vi "ArrDevMeasAction.vi"(6 "Scan":bool, 7 "DevId":i32, 8 "error in (no error)":errorcluster caption="entrée d'erreur (pas d'erreur)", 9 "CurvePointIndex":i32, 10 "AllPointIndex":i32, 11 "Device In":refnum<class "AndorSpectro.lvclass"> caption="DNL_LabVIEW Object in") -> (0 "error out":errorcluster caption="sortie d'erreur", 1 "ArrDevDat":T1[](array[typedef]), 2 "ArrDevDatOut":dbl[][](array[numeric]), 3 "Device Out":refnum<class "AndorSpectro.lvclass"> caption="DNL_LabVIEW Object out", 5 "MeasOut":dbl[](array[numeric]))   [LabVIEW 2019, in "AndorSpectro.lvclass"]
uses:
  AndorSpectro.lvclass
  C:/Programmes Labview/LabscanV1A/DevicesClass/BaseDevice/BaseDevice.lvclass
  Experiment Class/ArrDevData.ctl
  AndorSpectro.lvclass/AndorSpectro.ctl
  BaseDevice/BaseDevice.lvclass/BaseDevice.ctl
  <userlib>/ATSpectrograph/GUI/AndorNoiseCorr.ctl
  BaseDevice/Accessor/GetBaseDataPath.vi
  <userlib>/GenProg/ReadValByRefVariant.vi
  <userlib>/GenProg/ReadbyWeakRefBool.vi
  <userlib>/GenProg/ReadValByRefBool.vi
  <userlib>/GenProg/ReadValByRefDblArr.vi
  <userlib>/GenProg/ReadValByRefI32Arr2D.vi
panel:
  out "ControlsNames":string[](array[string])
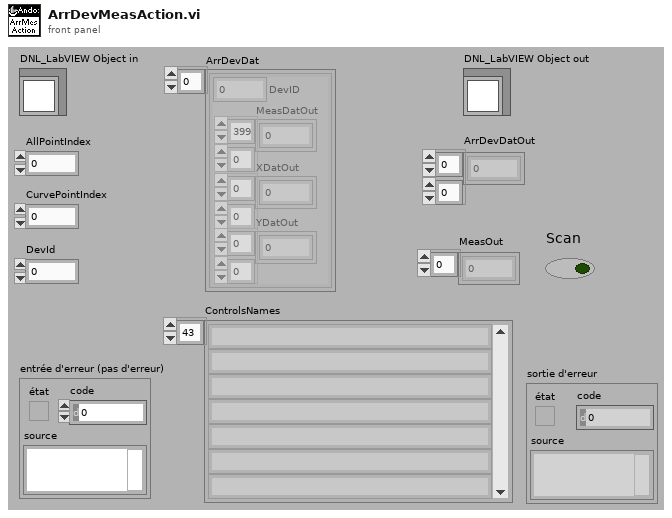
[diagram p1: front panel]
types:
  T1 = typedef "ArrDevData.ctl" = cluster{"MeasDatOut":dbl[][], "XDatOut":dbl[][], "YDatOut":dbl[][], "DevID":i32}
  T2 = typedef "AndorNoiseCorr.ctl" = enum16{"Off", "Selected Curve", "One For Every Acq"}
  T3 = cluster{"WB Start":i32, "WB End":i32, "Active":bool}[]
  T4 = cluster{"Message":string, "Data":variant, "Code":i32}
  T5 = typedef "AndorSpectro.lvclass/AndorSpectro_Func.ctl" = enum16{"ReadSpectrum (cnt)", "SetWavelenght (nm)"}
  T6 = cluster{"Scan":bool, "CurvePointIndex":i32, bool}
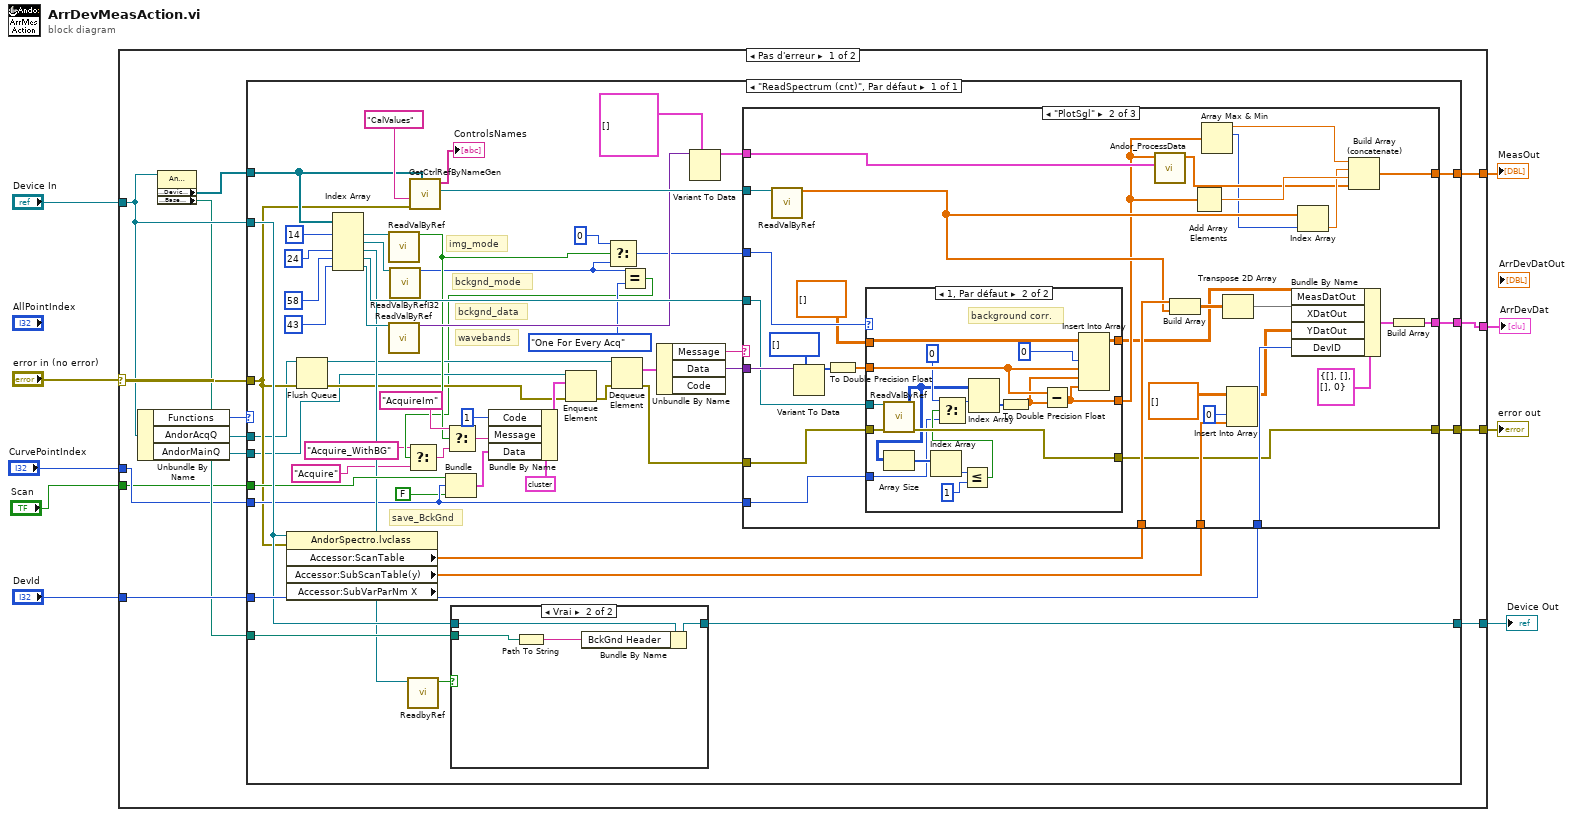
[diagram p0: block diagram]
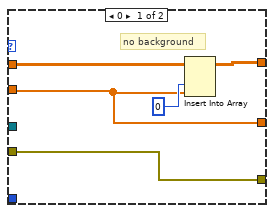
[diagram p4: hidden frame]
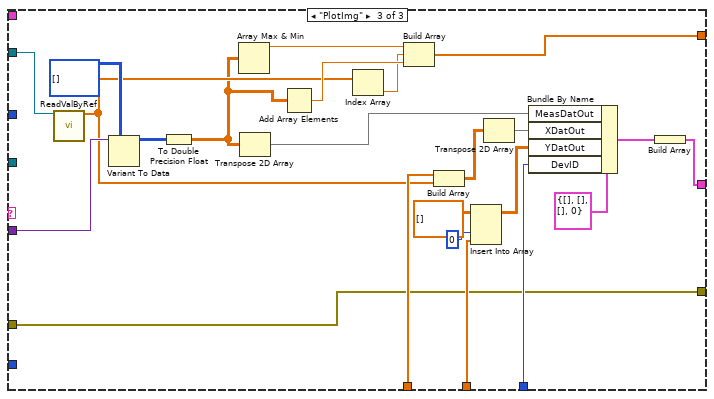
[diagram p5: hidden frame]
diagram:
  n1 = case shown="Pas d'erreur" "error in (no error)" {
    selector: "error in (no error)" -> [w22 w162]
    tunnel: [w12 w163] -> w8
    tunnel: "Device In" -> [w17 w163]
    tunnel: [w21 w162] -> w6
    tunnel: [w20 _] -> w5
    tunnel: "DevId" -> [w19 _]
    tunnel: [w15 _] -> w3
    tunnel: "CurvePointIndex" -> [w11 _]
    tunnel: "Scan" -> [w10 _]
    frame No Error {
      n2 = Unbundle By Name(w17) -> ("Functions"=w23:T5, "AndorAcqQ"=w18:refnum<queue>, "AndorMainQ"=w14:refnum<queue>)
      n3 = property class="AndorSpectro.lvclass"(reference=w17) -> ("Accessor:DeviceCtrl"=w16:refnum<vi>[], "Accessor:BaseDataPath"=w13:path)  [unwired: 1 in, 2 out]
      n4 = case shown="\"ReadSpectrum (cnt)\", Par défaut" w23 {
        tunnel: w22 -> [w35]
        tunnel: [w55] -> w21
        tunnel: w17 -> [w61]
        tunnel: [w77] -> w20
        tunnel: w19 -> [w76]
        tunnel: w18 -> [w34]
        tunnel: w16 -> [w65]
        tunnel: [w72] -> w15
        tunnel: w14 -> [w28]
        tunnel: w13 -> [w62]
        tunnel: [w60] -> w12
        tunnel: w11 -> [w39]
        tunnel: w10 -> [w45]
        frame "ReadSpectrum (cnt)", Default {
          # "wavebands"
          # "bckgnd_data"
          # "save_BckGnd"
          # "bckgnd_mode"
          # "img_mode"
          n5 = property class="AndorSpectro.lvclass" props=["Accessor:ScanTable", "Accessor:SubScanTable(y)", "Accessor:SubVarParNm X"](reference=w61, error in=w35) -> ("Accessor:ScanTable"=w40:dbl[], "Accessor:SubScanTable(y)"=w73:dbl[])  [unwired: 3 out]
          n6 = Flush Queue(queue=w34, error in (no error)=w35) -> (queue out=w32:refnum<queue>, error out=w33:errorcluster)  [unwired: 1 out]
          n7 = Index Array(array=w65, index #1=14 ("indice"), index #3=24 ("indice"), index #4=58 ("indice"), index #5=43 ("indice")) -> (element #1=w51:refnum<vi>, element #2=w41:refnum<vi>, element #3=w42:refnum<vi>, element #4=w57:refnum<vi>, element #5=w50:refnum<vi>)  [unwired: 1 in]
          n8 = call-poly <userlib>:"ReadValByRef.vi"("Control Ref"=w51) -> ("Valeur"=w38:bool)  [unwired: 13 in, 1 out]
          n9 = call-poly <userlib>:"ReadValByRef.vi"("Control Ref"=w50) -> ("Valeur"=w49:variant)  [unwired: 13 in, 1 out]
          n10 = call <userlib>:"ReadValByRefI32.vi"("Control Ref"=w41) -> ("Valeur"=w29:i32)  [unwired: 13 in, 1 out]
          n11 = call-poly <userlib>:"ReadbyRef.vi"("Control Ref"=w42) -> ("Valeur"=w59:bool)  [unwired: 9 in, 1 out]
          n12 = call <userlib>:"GetCtrlRefByNameGen.vi"("Commandes []"=w65, "ErrorIn(No Error)"=w35, "ControlName"="CalValues") -> ("ControlsRefs"=w66:refnum<vi>, "ControlsNames"=→"ControlsNames":string[])  [unwired: 6 in, 1 out]
          n13 = Bundle("Scan"=w45, "CurvePointIndex"=w39, FALSE) -> (w44:T6)  [unwired: 1 in]
          n14 = case shown="Vrai" w59 {
            tunnel: w62 -> [_ w80]
            tunnel: w61 -> [w78 w82]
            tunnel: [w78 w81] -> w60
            frame False {
            }
            frame True {
              n15 = Path To String(path=w80) -> (string=w79:string)
              n16 = Bundle By Name(cluster=w82, "BckGnd Header"=w79) -> (w81:refnum<class "AndorSpectro.lvclass">)
            }
          }
          n17 = Select(t=0 ("cas vrai"), s=w38, f=w29) -> (s? t:f=w37:i32)
          n18 = Equal?(x=w29, y=AndorNoiseCorr."One For Every Acq" ("Backgnd Mode")) -> (x = y?=w26:bool)
          n19 = Select(t="Acquire_WithBG", s=w26, f="Acquire" ("Message")) -> (s? t:f=w27:string)
          n20 = Select(t="AcquireIm" ("Message"), s=w38, f=w27) -> (s? t:f=w53:string)
          n21 = Bundle By Name(cluster=T4 {"Message"="", "Data"=variant, "Code"=0} ("élément"), "Code"=1, "Message"=w53, "Data"=w44) -> (w71:T4)
          n22 = Enqueue Element(queue=w28, element=w71, error in (no error)=w33) -> (error out=w70:errorcluster)  [unwired: 1 in, 2 out]
          n23 = Dequeue Element(queue=w32, error in (no error)=w70) -> (element=w75:T4, error out=w56:errorcluster)  [unwired: 1 in, 2 out]
          n24 = Unbundle By Name(w75) -> ("Message"=w68:string, "Data"=w74:variant)  [unwired: 1 out]
          n25 = Variant To Data(type=T3 [] ("WaveBands"), Variant=w49) -> (data=w47:T3)  [unwired: 1 in, 1 out]
          n26 = case shown="\"PlotSgl\"" w68 {
            tunnel: [_ w113 w159] -> w77
            tunnel: w76 -> [_ w112 w158]
            tunnel: w74 -> [_ w109 w155]
            tunnel: w73 -> [_ w96 w143]
            tunnel: [_ w106 w152] -> w72
            tunnel: w40 -> [_ w102 w148]
            tunnel: w66 -> [_ w101 w147]
            tunnel: w57 -> [_ w95 _]
            tunnel: w56 -> [w83 w94 w139]
            tunnel: [w83 w93 w139] -> w55
            tunnel: w37 -> [_ w92 _]
            tunnel: w47 -> [_ w91 _]
            tunnel: w39 -> [_ w84 _]
            frame Default {
            }
            frame "PlotSgl" {
              n27 = call-poly <userlib>:"ReadValByRef.vi"("Control Ref"=w101) -> ("Valeur"=w100:dbl[])  [unwired: 13 in, 1 out]
              n28 = Variant To Data(type=i32[] [] ("Data out"), Variant=w109) -> (data=w110:i32[])  [unwired: 1 in, 1 out]
              n29 = To Double Precision Float(number=w110) -> (double precision float=w88:dbl[])
              n30 = case shown="1, Par défaut" w92 {
                tunnel: w95 -> [_ w138]
                tunnel: w94 -> [w120 w137]
                tunnel: [w120 w136] -> w93
                tunnel: [w117 w130] -> w90
                tunnel: w88 -> [w117 w132]
                tunnel: [w119 w133] -> w87
                tunnel: dbl[][] [] ("tableau") -> [w116 w134]
                tunnel: w84 -> [_ w124]
                frame 0 {
                  # "no background"
                  n31 = Insert Into Array(array=w116, index (col)=0 ("indice désactivé (col)"), new element=w117) -> (w119:dbl[][])  [unwired: 1 in]
                }
                frame 1, Default {
                  # "background corr."
                  n32 = call-poly <userlib>:"ReadValByRef.vi"("Control Ref"=w138, "error in"=w137) -> ("Valeur"=w121:i32[][], "error out"=w136:errorcluster)  [unwired: 12 in]
                  n33 = Array Size(array=w121) -> (size(s)=w128:i32[])
                  n34 = Index Array(array=w128) -> (element=w127:i32)  [unwired: 1 in]
                  n35 = Less Or Equal?(x=w127, y=1) -> (x <= y?=w125:bool)
                  n36 = Select(t=0 ("cas vrai"), s=w125, f=w124) -> (s? t:f=w122:i32)
                  n37 = Index Array(array=w121, index (row)=w122) -> (element=w129:i32[])  [unwired: 1 in]
                  n38 = To Double Precision Float(number=w129) -> (double precision float=w131:dbl[])
                  n39 = Subtract(x=w132, y=w131) -> (x-y=w130:dbl[])
                  n40 = Insert Into Array(array=w134, index (col)=0 ("indice désactivé (col)"), new element #1=w132, new element #2=w131, new element #3=w130) -> (w133:dbl[][])  [unwired: 1 in]
                }
              }
              n41 = call <userlib>:"Andor_ProcessData.vi"("WaveBands"=w91, "Data"=w90) -> ("WB Cnts"=w89:dbl[])  [unwired: 8 in, 1 out]
              n42 = Build Array(w102, w100) -> (w108:dbl[][])
              n43 = Add Array Elements(numeric array=w90) -> (sum=w105:dbl)
              n44 = Array Max & Min(array=w90) -> (max value=w107:dbl, max index (indices)=w85:i32)  [unwired: 2 out]
              n45 = Transpose 2D Array(2D array=w108) -> (transposed array=w103:dbl[][])
              n46 = Insert Into Array(array=dbl[][] [] ("tableau"), index (col)=0 ("taille de la dimension"), new element=w96) -> (w97:dbl[][])  [unwired: 1 in]
              n47 = Bundle By Name(cluster=T1 {"MeasDatOut"=[], "XDatOut"=[], "YDatOut"=[], "DevID"=0} ("cluster de sortie"), "MeasDatOut"=w87, "XDatOut"=w103, "YDatOut"=w97, "DevID"=w112) -> (w114:T1)
              n48 = Index Array(array=w100, index=w85) -> (element=w104:dbl)
              n49 = Build Array (concatenate)(w107, w104, w105, w89) -> (w106:dbl[])
              n50 = Build Array(w114) -> (w113:T1[])
            }
            frame "PlotImg" {
              n51 = call-poly <userlib>:"ReadValByRef.vi"("Control Ref"=w147) -> ("Valeur"=w146:dbl[])  [unwired: 13 in, 1 out]
              n52 = Variant To Data(type=i32[][] [] ("Data out"), Variant=w155) -> (data=w156:i32[][])  [unwired: 1 in, 1 out]
              n53 = To Double Precision Float(number=w156) -> (double precision float=w145:dbl[][])
              n54 = Array Max & Min(array=w145) -> (max value=w153:dbl)  [unwired: 3 out]
              n55 = Transpose 2D Array(2D array=w145) -> (transposed array=w144:dbl[][])
              n56 = Add Array Elements(numeric array=w145) -> (sum=w151:dbl)
              n57 = Index Array(array=w146) -> (element=w150:dbl)  [unwired: 1 in]
              n58 = Build Array(w153, w150, w151) -> (w152:dbl[])
              n59 = Build Array(w148, w146) -> (w154:dbl[][])
              n60 = Insert Into Array(array=dbl[][] [] ("tableau"), index (col)=0 ("taille de la dimension"), new element=w143) -> (w140:dbl[][])  [unwired: 1 in]
              n61 = Transpose 2D Array(2D array=w154) -> (transposed array=w149:dbl[][])
              n62 = Bundle By Name(cluster=T1 {"MeasDatOut"=[], "XDatOut"=[], "YDatOut"=[], "DevID"=0} ("cluster de sortie"), "MeasDatOut"=w144, "XDatOut"=w149, "YDatOut"=w140, "DevID"=w158) -> (w160:T1)
              n63 = Build Array(w160) -> (w159:T1[])
            }
          }
        }
      }
    }
    frame Error {
    }
  }
  "error out" <- w6
  "Device Out" <- w8
  "ArrDevDat" <- w5
  "MeasOut" <- w3
